vi "DateTimeOffset for MS SQL.vi"() -> (2 "date/time string":string)   [LabVIEW 2016, in "MS SQL Saver.lvlib"]
uses:
  Focal Point End Of Line Tester/MS SQL Saver/MS SQL Saver.lvlib
panel:
  out "match substring":string
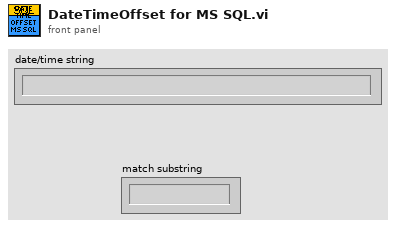
[diagram p1: front panel]
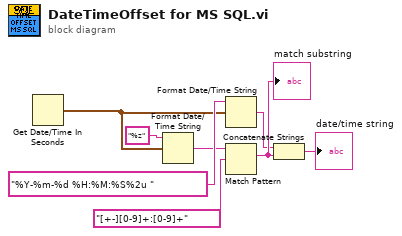
[diagram p0: block diagram]
diagram:
  n1 = Get Date/Time In Seconds() -> (seconds since 1Jan1904=w7:timestamp)
  n2 = Format Date/Time String(time format string (%c)="%z", seconds (now)=w7) -> (date/time string=w5:string)  [unwired: 1 in]
  n3 = Format Date/Time String(time format string (%c)="%Y-%m-%d %H:%M:%S%2u ", seconds (now)=w7) -> (date/time string=w2:string)  [unwired: 1 in]
  n4 = Match Pattern(string=w5, regular expression="[+-][0-9]+:[0-9]+") -> (match substring=w3:string)  [unwired: 1 in, 3 out]
  "match substring" <- w3
  n5 = Concatenate Strings(w2, w3) -> (→"date/time string":string)
